vi "Decimal to Binary Converter.vi"() -> ()   [LabVIEW 2009]
panel:
  out "Binary Output":bool[](array[boolean])
  in  "Decimal input":u8[](array[numeric])
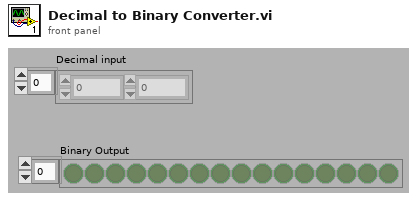
[diagram p1: front panel]
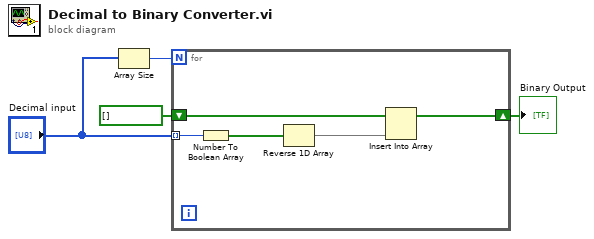
[diagram p0: block diagram]
diagram:
  n1 = Array Size(array="Decimal input") -> (size(s)=w4:i32)
  n2 = for {
    N: w4 -> [_]
    shift-right: [w5] -> w1
    shift-left: bool[] [] -> [w6]
    tunnel: "Decimal input" -> [w9] mode=indexing
    n3 = Number To Boolean Array(number=w9) -> (Boolean array=w8:bool[])
    n4 = Reverse 1D Array(array=w8) -> (reversed array=w7:bool[])
    n5 = Insert Into Array(array=w6, new element=w7) -> (w5:bool[])  [unwired: 1 in]
  }
  "Binary Output" <- w1
